vi "Read Data.vi"(8 "error in (no error)":errorcluster, 11 "IPS120 in":refnum<class "IPS120.lvclass">) -> (0 "error out":errorcluster, 2 "Data":waveform(dbl)[](array[waveform]), 3 "IPS120 out":refnum<class "IPS120.lvclass">)   [LabVIEW 2015, in "IPS120.lvclass"]
uses:
  IPS120.lvclass
  ITC503/Controls/ITC503 FP Data.ctl
  OO Devices/Device/Read Controls Snapshot.vi
  Instrument/Read VISA Resource.vi
  OO Devices/Device/Read Control Panel Loaded.vi
  Instrument/Write VISA Resource.vi
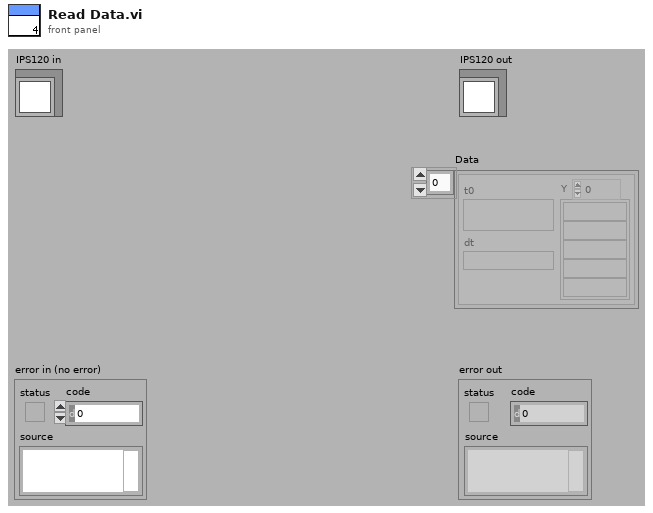
[diagram p1: front panel]
types:
  T1 = typedef "ITC503 FP Data.ctl" = cluster{"Channels to measure":i32[]}
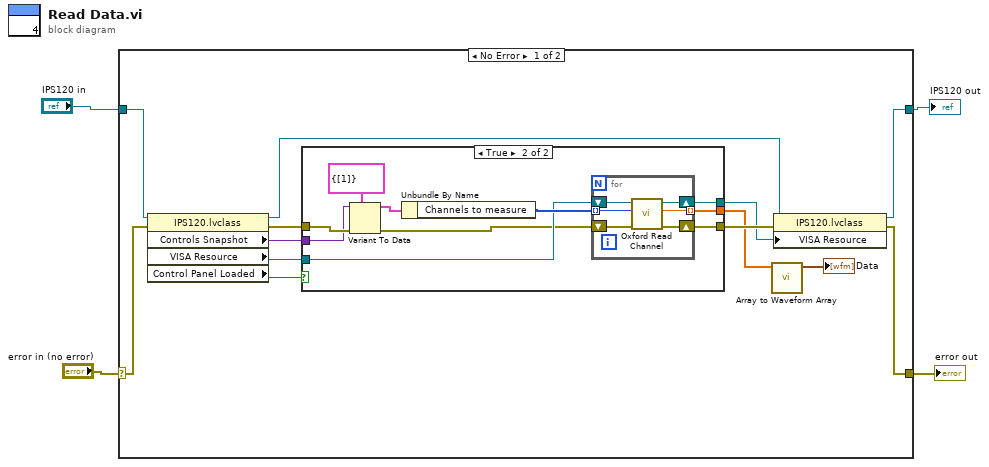
[diagram p0: block diagram]
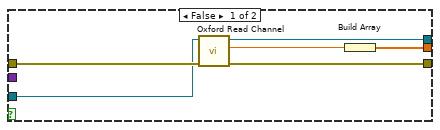
[diagram p2: hidden frame]
diagram:
  n1 = case shown="No Error" "error in (no error)" {
    selector: "error in (no error)" -> [w8 w41]
    tunnel: [w5 w41] -> w3
    tunnel: [w6 w40] -> w1
    tunnel: "IPS120 in" -> [w7 w40]
    frame No Error {
      n2 = property class="IPS120.lvclass"(reference=w7, error in=w8) -> (reference out=w10:refnum<class "IPS120.lvclass">, error out=w15:errorcluster, "Controls Snapshot"=w14:variant, "VISA Resource"=w11:refnum<visa-resource-name>, "Control Panel Loaded"=w9:bool)
      n3 = case shown="True" w9 {
        tunnel: [w22 w33] -> w17
        tunnel: w15 -> [w23 w32]
        tunnel: w14 -> [_ w31]
        tunnel: [w19 w28] -> w13
        tunnel: [w18 w26] -> w12
        tunnel: w11 -> [w21 w25]
        frame False {
          n4 = call "Oxford Read Channel.vi"("error in (no error)"=w23, "VISA resource name"=w21) -> ("error out"=w22:errorcluster, "Data"=w20:dbl, "VISA resource name out"=w18:refnum<visa-resource-name>)  [unwired: 6 in, 1 out]
          n5 = Build Array(w20) -> (w19:dbl[])
        }
        frame True {
          n6 = Variant To Data(error in=w32, type=T1 {"Channels to measure"=[1]} ("Data"), Variant=w31) -> (data=w29:T1, error out=w24:errorcluster)
          n7 = Unbundle By Name(w29) -> ("Channels to measure"=w27:i32[])
          n8 = for {
            tunnel: [w35] -> w28 mode=indexing
            shift-right: [w36] -> w33
            shift-left: w24 -> [w38]
            tunnel: w27 -> [w34] mode=indexing
            shift-right: [w37] -> w26
            shift-left: w25 -> [w39]
            n9 = call "Oxford Read Channel.vi"("error in (no error)"=w38, "Channel #"=w34, "VISA resource name"=w39) -> ("error out"=w36:errorcluster, "Data"=w35:dbl, "VISA resource name out"=w37:refnum<visa-resource-name>)  [unwired: 5 in, 1 out]
          }
        }
      }
      n10 = call "Array to Waveform Array.vi"("Array"=w13) -> ("Waveform"=→"Data":waveform(dbl)[])  [unwired: 10 in]
      n11 = property class="IPS120.lvclass"(reference=w10, error in=w17, "VISA Resource"=w12) -> (reference out=w6:refnum<class "IPS120.lvclass">, error out=w5:errorcluster)
    }
    frame Error {
    }
  }
  "error out" <- w3
  "IPS120 out" <- w1
